vi "LVClass_Camera get background.vi"(0 "Camera in":refnum<class "Camera.lvclass">, 5 "BG Image IN":refnum<class "Image.lvclass">, 11 "error in (no error)":errorcluster) -> (4 "Camera out":refnum<class "Camera.lvclass">, 6 "BG Image OUT":refnum<class "Image.lvclass">, 15 "error out":errorcluster)   [LabVIEW 2020, in "Camera.lvclass"]
doc: "Get camera parameters which are gettable and settable parameter \n\n<B>CameraIn</B> : Camera object.\n<B>CameraOut</B> : Camera object.\n<B>BG Image IN</B> : Image object to store the defined background image object if it is allready defined throught camera object method \"LVClass_Camera set background.vi\".\n<B>BG Image OUT</B> : Image object to store the defined background image"
uses:
  Camera.lvclass
  Image.lvclass
  Camera.lvclass/Camera.ctl
  LVClass_Image read Image Compat ptr.vi
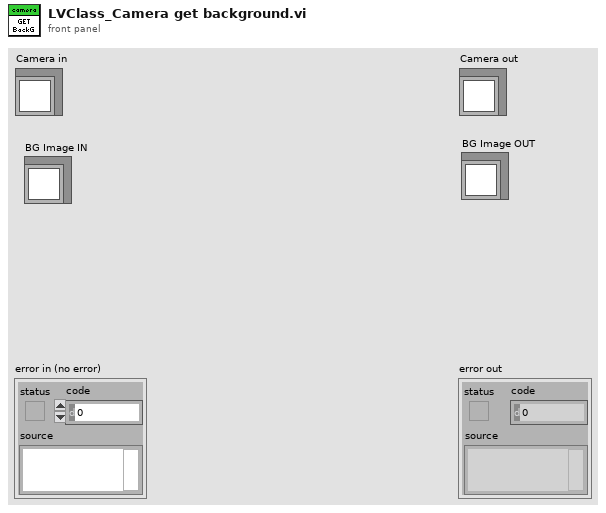
[diagram p1: front panel]
types:
  T1 = typedef "ClassID.ctl" = i64
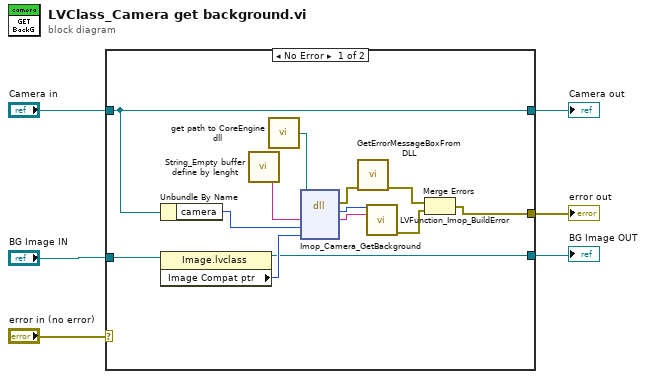
[diagram p0: block diagram]
diagram:
  n1 = case shown="No Error" "error in (no error)" {
    selector: "error in (no error)" -> [_ w22]
    tunnel: [w7 w22] -> w5
    tunnel: [w11 w21] -> w3
    tunnel: "Camera in" -> [w11 w21]
    tunnel: [w12 w20] -> w2
    tunnel: "BG Image IN" -> [w14 w20]
    frame No Error {
      n2 = Unbundle By Name(w11) -> ("camera"=w10:T1)
      n3 = property class="Image.lvclass"(reference=w14) -> (reference out=w12:refnum<class "Image.lvclass">, "Image Compat ptr"=w13:T1)  [unwired: 1 in, 1 out]
      n4 = call "String_Empty buffer define by lenght.vi"() -> ("Empty buffer"=w19:string)  [unwired: 1 in]
      n5 = call "get path to CoreEngine dll.vi"() -> ("path to wavekit library"=w16:path)  [unwired: 14 in, 1 out]
      n6 = dll-call lib="D:/2_trunk/Soft_haso/ImOpCoreEngine4_LV2011/DLLs/ImopEngine4_vc100.dll" fn="Imop_Camera_GetBackground"(path in=w16, "message"=w19, "camera"=w10, "HASO_image"=w13) -> (error out=w15:errorcluster, "return type"=w18:i32, "message"=w17:string)  [unwired: 4 in, 1 out]
      n7 = call "GetErrorMessageBoxFromDLL.vi"("error IN"=w15) -> ("error OUT"=w9:errorcluster)  [unwired: 10 in]
      n8 = call "LVFunction_Imop_BuildError.vi"("code"=w18, "String to Prepend to source (\"\")"=w17) -> ("error out"=w8:errorcluster)  [unwired: 13 in]
      n9 = Merge Errors(w9, w8) -> (w7:errorcluster)
    }
    frame Error {
    }
  }
  "error out" <- w5
  "Camera out" <- w3
  "BG Image OUT" <- w2
